vi "Set Server State UE.vi"(10 "Server State UE":refnum<user-event>, 11 "OOP Query Server in":refnum<class "OOP Query Server.lvclass">) -> (3 "OOP Query Server out":refnum<class "OOP Query Server.lvclass">)   [LabVIEW 2019, in "OOP Query Server.lvlib" / "OOP Query Server.lvclass"]
uses:
  OOP Query Server.lvclass
  typeDefs/Server State Data.ctl
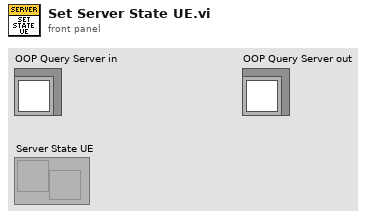
[diagram p1: front panel]
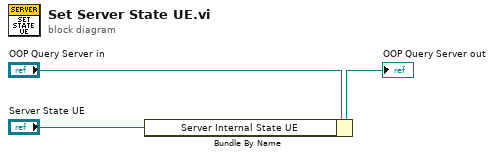
[diagram p0: block diagram]
diagram:
  n1 = Bundle By Name(cluster="OOP Query Server in", "Server Internal State UE"="Server State UE") -> (→"OOP Query Server out":refnum<class "OOP Query Server.lvclass">)
